vi "SendTcpStartCommand.vi"(6 "機器番号":u8, 11 "アドレス":string) -> (1 "送信文字列":string, 2 "空?":bool, 3 "Send List Out":cluster{"Address":string, "Data":string}[](array[cluster]))   [LabVIEW 2017]
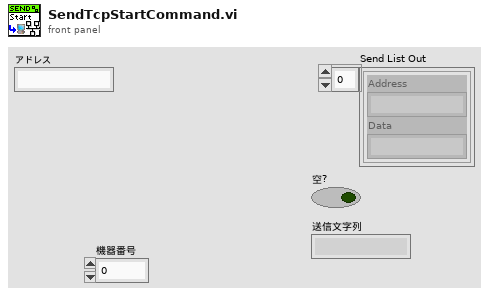
[diagram p1: front panel]
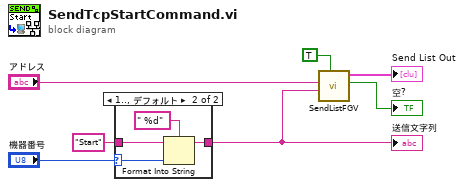
[diagram p0: block diagram]
diagram:
  n1 = case shown="1.., デフォルト" "機器番号" {
    selector: "機器番号" -> [_ w10]
    tunnel: [w8 w12] -> w7
    tunnel: "Start" ("要素") -> [w8 w9]
    frame 0 {
    }
    frame 1.., Default {
      n2 = Format Into String(format string=" %d" ("形式文字列"), initial string=w9, w10) -> (resulting string=w12:string)  [unwired: 1 in, 1 out]
    }
  }
  "送信文字列" <- w7
  n3 = call "SendListFGV.vi"("Set"=TRUE, "Data"=w7, "アドレス"="アドレス") -> ("空?"=→"空?":bool, "Send List Out"=→"Send List Out":cluster{"Address":string, "Data":string}[])  [unwired: 6 in, 1 out]
